vi "BB_Rectangle_edge_discriminator.vi"(9 "Cluster":T1, 10 "X Resolution":i32, 11 "Y Resolution":i32) -> (3 "Edge":bool)   [LabVIEW 2012]
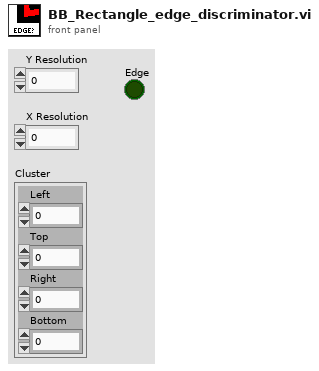
[diagram p1: front panel]
types:
  T1 = cluster{"Left":dbl, "Top":dbl, "Right":dbl, "Bottom":dbl}
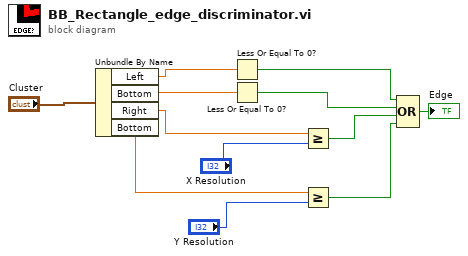
[diagram p0: block diagram]
diagram:
  n1 = Unbundle By Name("Cluster") -> ("Left"=w11:dbl, "Bottom"=w10:dbl, "Right"=w9:dbl, "Bottom"=w7:dbl)
  n2 = Less Or Equal To 0?(x=w11) -> (x <= 0?=w5:bool)
  n3 = Less Or Equal To 0?(x=w10) -> (x <= 0?=w4:bool)
  n4 = Greater Or Equal?(x=w9, y="X Resolution") -> (x >= y?=w3:bool)
  n5 = Greater Or Equal?(x=w7, y="Y Resolution") -> (x >= y?=w2:bool)
  n6 = Compound Arithmetic op=OR(w5, w4, w3, w2) -> (→"Edge":bool)
